vi "getData.vi"(8 "error in":T1, 9 "fullOnly":bool, 10 "length":i32, 11 "Channel":i32) -> (0 "error out":T1, 2 "Spec_Array":cluster{sgl[], "specArrayY_bwd":sgl[]}[](array[cluster]), 3 "scanData":sgl[][][](array[numeric]), 4 "unitStrVal":string, 6 "unitStrXY":string)   [LabVIEW 2016]
doc: "Processes the data that is retrieved over a registered channel and has the corresponding data arrays as outputs.\nUse the getDataLine.vi instead of this VI to access data from the LineVIEW.\nFor a detailed description of the inputs and outputs please refer to the ASC500 manual Remote Control."
uses:
  Controls/Error_Out.ctl
  Files_ASC500/DLL/ASC500_RemoteControlV27.dll
panel:
  out "mar":i32[](array[numeric])
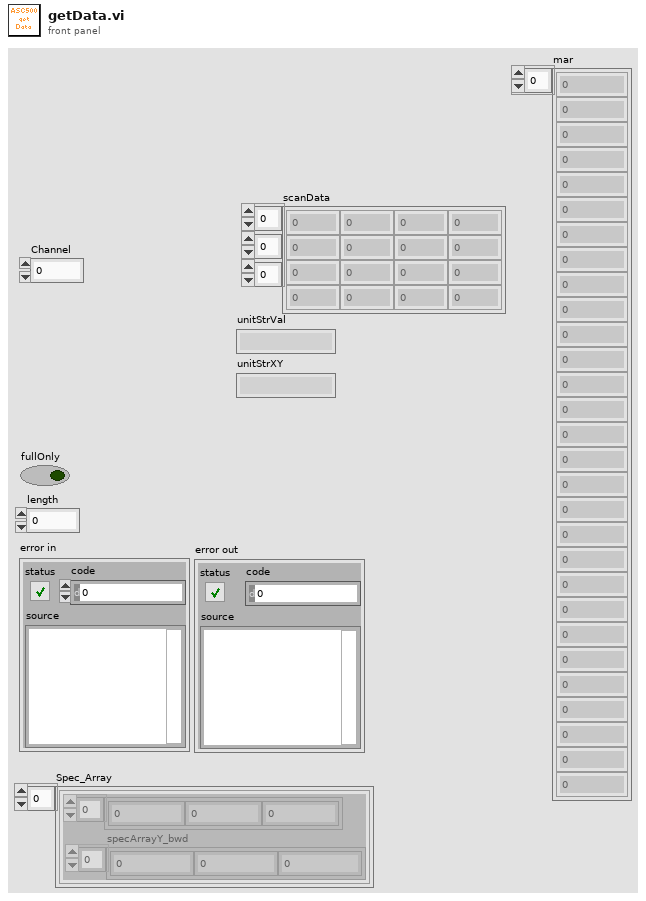
[diagram p1: front panel]
types:
  T1 = typedef "Error_Out.ctl" = errorcluster
  T2 = cluster{"specArrayX":sgl[], "specArrayY_fwd":sgl[]}
  T3 = cluster{"specArrayX":sgl[], "specArrayY_bwd":sgl[]}
  T4 = cluster{"specArrayX":sgl[], "specArrayY_bwd":sgl[]}[]
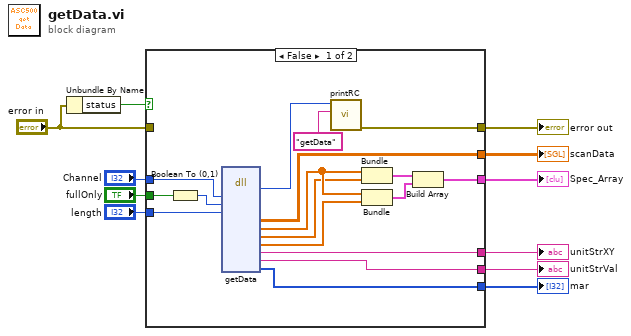
[diagram p0: block diagram]
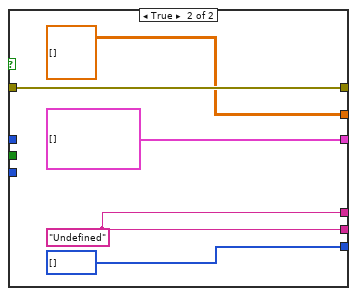
[diagram p2: hidden frame]
diagram:
  n1 = Unbundle By Name("error in") -> ("status"=w5:bool)
  n2 = case shown="False" w5 {
    tunnel: "error in" -> [_ w33]
    tunnel: [w27 w33] -> w4
    tunnel: "Channel" -> [w25 _]
    tunnel: "fullOnly" -> [w24 _]
    tunnel: "length" -> [w22 _]
    tunnel: [w12 w29] -> w2
    tunnel: [w13 w29] -> w1
    tunnel: [w19 cluster{sgl[], "specArrayY_bwd":sgl[]}[] []] -> w9
    tunnel: [w18 i32[] [] ("mar")] -> w10
    tunnel: [w17 sgl[][][] [] ("scanData")] -> w11
    frame False {
      n3 = Boolean To (0,1)(Boolean=w24) -> (0, 1=w23:i16)
      n4 = dll-call lib="G:/SCMOperations/Share/ELE/Produkt Information/ASC500/04 Remote Control/02 development versions/2018Nov06/Files_ASC500/DLL/ASC500_RemoteControlV27.dll" fn="getData"("channel"=w25, "fullOnly"=w23, "length"=w22) -> ("RC"=w26:u32, "scanData"=w17:sgl[][][], "specArrayX"=w16:sgl[], "specArrayY_fwd"=w15:sgl[], "specArrayY_bwd"=w14:sgl[], "unitStrXY"=w13:string, "unitStrVal"=w12:string, "mar"=w18:i32[])  [unwired: 13 in, 2 out]
      n5 = call "printRC.vi"("additional information"="getData", "RC"=w26) -> ("error out"=w27:T1)  [unwired: 9 in]
      n6 = Bundle("specArrayX"=w16, "specArrayY_fwd"=w15) -> (w21:T2)  [unwired: 1 in]
      n7 = Bundle("specArrayX"=w16, "specArrayY_bwd"=w14) -> (w20:T3)  [unwired: 1 in]
      n8 = Build Array(w21, w20) -> (w19:T4)
    }
    frame True {
      w29 = "Undefined" ("unitStrVal")
    }
  }
  "error out" <- w4
  "Spec_Array" <- w9
  "mar" <- w10
  "scanData" <- w11
  "unitStrVal" <- w2
  "unitStrXY" <- w1
